vi "Emballage_BDD_lectureSQL_V_LIGCDECLTVAL.vi"(8 "Error in":errorcluster caption="Error in (no error)", 11 "NO_CDEVAL":string) -> (0 "Error out":errorcluster, 1 "CMD_DejaBoucle?":bool, 2 "Erreur de  comunication":bool, 3 "Donnees":string[][](array[string]))   [LabVIEW 2020]
uses:
  Modules/FS/60_FS_Controles/60_FS_SetGet.ctl
  <vilib>/addons/database/Connection.llb/DB Tools Open Connec (Path).vi
  <vilib>/addons/database/Connection.llb/Conn Execute.vi
  <vilib>/addons/database/Recordset.llb/Rec Fetch Recordset Data (R).vi
  <vilib>/addons/database/Recordset.llb/Rec Destroy - Connection.vi
  <vilib>/addons/database/NI_Database_API.lvlib
panel:
  out "temps_sec":dbl
  out "CMD_interne?":bool
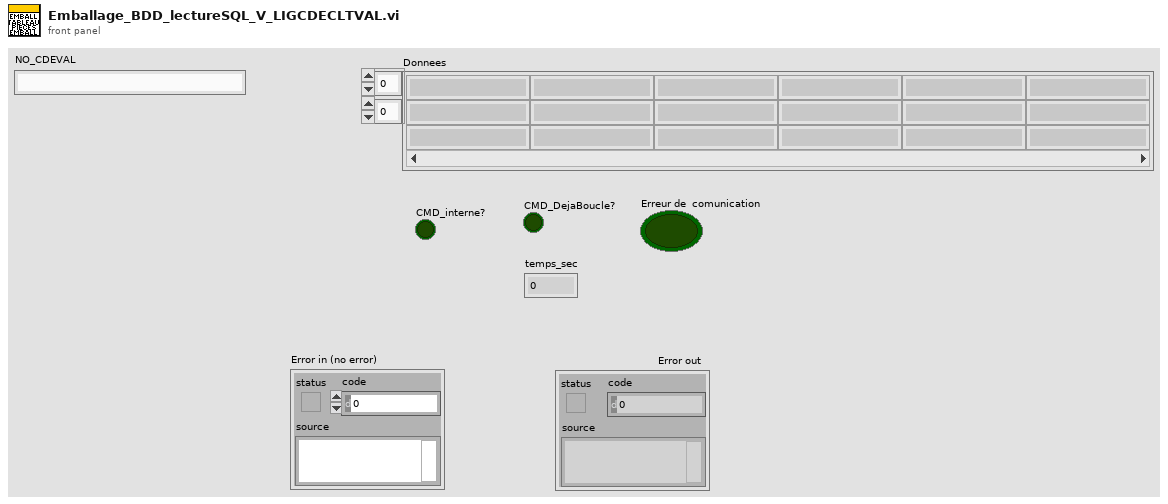
[diagram p1: front panel]
types:
  T1 = typedef "60_FS_SetGet.ctl" = enum16{"set", "get"}
  T2 = typedef "60_FS_CLT_Chemins.ctl" = cluster{"Racine_local":path, "Racine_reseau":path, "Racine_Support_Application":path, "Fichier_Journalisation":path, "Connexion_BDD_VSX":path, "Connexion_BDD_PLZ":path}
  T3 = typedef "NI_Database_API.lvlib/Conn ObjectReference.ctl" = refnum<k1>
  T4 = typedef "NI_Database_API.lvlib/Rec ObjectReference.ctl" = refnum<k1>
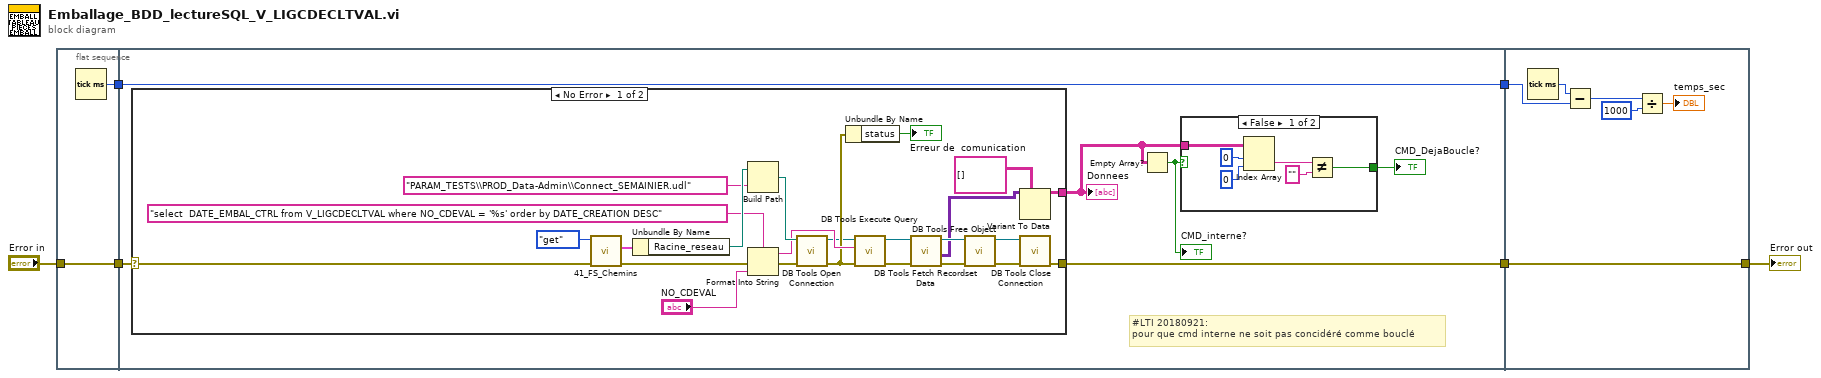
[diagram p0: block diagram]
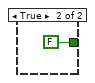
[diagram p2: hidden frame]
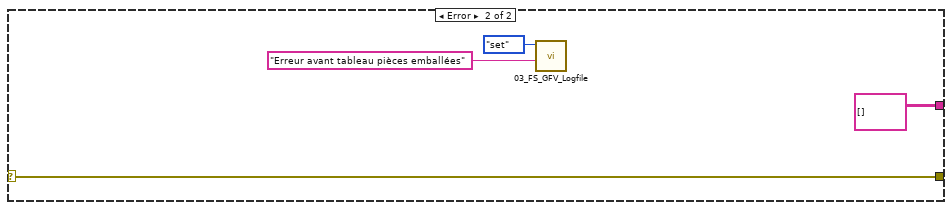
[diagram p3: hidden frame]
diagram:
  n1 = flat-sequence {
    tunnel: [w8] -> w6
    tunnel: "Error in" -> [w8]
    tunnel: [w7] -> w2
    tunnel: w6 -> [w11]
    tunnel: [w10] -> w4
    tunnel: w2 -> [w9]
    tunnel: [w9] -> w1
    tunnel: w4 -> [w55]
    tunnel: [w55] -> w3
    tunnel: w1 -> [w53]
    frame #0 {
      n2 = Tick Count (ms)() -> (millisecond timer value=w7:u32)
    }
    frame #1 {
      # "#LTI 20180921:\npour que cmd interne ne soit pas concidéré comme bouclé"
      n3 = case shown="No Error" w11 {
        selector: w11 -> [w39 w49]
        tunnel: [w38 w49] -> w10
        tunnel: [w31 string[][] [] ("Liste des champs à lire 2")] -> w12
        frame No Error {
          n4 = call "41_FS_Chemins.vi"("error in (no error)"=w39, "SetGet"=60_FS_SetGet."get") -> ("error out"=w40:errorcluster, "CLT_Chemins_out"=w42:T2)  [unwired: 8 in]
          n5 = Unbundle By Name(w42) -> ("Racine_reseau"=w29:path)
          n6 = Build Path(base path=w29, name or relative path="PARAM_TESTS\\PROD_Data-Admin\\Connect_SEMAINIER.udl" ("nom ou chemin relatif")) -> (appended path=w27:path)
          n7 = Format Into String(format string="select  DATE_EMBAL_CTRL from V_LIGCDECLTVAL where NO_CDEVAL = '%s' order by DATE_CREATION DESC" ("chaîne de format"), error in=w40, "NO_CDEVAL") -> (resulting string=w26:string, error out=w43:errorcluster)  [unwired: 1 in]
          n8 = call-poly <vilib>:"DB Tools Open Connection.vi"("error in (no error)"=w43, "connection information"=w27) -> ("error out"=w23:errorcluster, "connection reference"=w22:T3)  [unwired: 6 in]
          n9 = Unbundle By Name(w23) -> ("status"=→"Erreur de  comunication":bool)
          n10 = call-poly <vilib>:"DB Tools Execute Query.vi"("error in (no error)"=w23, "SQL query"=w26, "connection reference"=w22) -> ("error out"=w37:errorcluster, "recordset reference"=w35:T4)  [unwired: 5 in]
          n11 = call-poly <vilib>:"DB Tools Fetch Recordset Data.vi"("error in (no error)"=w37, "recordset reference"=w35) -> ("error out"=w36:errorcluster, "recordset data"=w33:variant[][], "recordset reference out"=w34:T4)  [unwired: 3 in]
          n12 = call-poly <vilib>:"DB Tools Free Object.vi"("error in (no error)"=w36, "recordset reference"=w34) -> ("error out"=w45:errorcluster, "connection reference"=w44:T3)  [unwired: 8 in]
          n13 = Variant To Data(type=string[][] [] ("Liste des champs à lire 2"), Variant=w33) -> (data=w31:string[][])  [unwired: 1 in, 1 out]
          n14 = call <vilib>:"DB Tools Close Connection.vi"("error in (no error)"=w45, "connection reference"=w44) -> ("error out"=w38:errorcluster)  [unwired: 5 in]
        }
        frame Error {
          n15 = call "03_FS_GFV_Logfile.vi"("Chaîne"="Erreur avant tableau pièces emballées", "States"=60_FS_SetGet."set") -> ()  [unwired: 8 in, 2 out]
        }
      }
      "Donnees" <- w12
      n16 = Empty Array?(array=w12) -> (empty?=w14:bool)
      "CMD_interne?" <- w14
      n17 = case shown="False" w14 {
        tunnel: [w16 FALSE] -> w13
        tunnel: w12 -> [w20 _]
        frame False {
          n18 = Index Array(array=w20, index (row)=0 ("indice (ligne)"), index (col)=0 ("indice désactivé (col)")) -> (element=w18:string)
          n19 = Not Equal?(x=w18, y="") -> (x != y?=w16:bool)
        }
        frame True {
        }
      }
      "CMD_DejaBoucle?" <- w13
    }
    frame #2 {
      n20 = Tick Count (ms)() -> (millisecond timer value=w54:u32)
      n21 = Subtract(x=w54, y=w53) -> (x-y=w52:u32)
      n22 = Divide(x=w52, y=u32 1000) -> (x/y=→"temps_sec":dbl)
    }
  }
  "Error out" <- w3
